vi "Filter Error Codes.vi"   [LabVIEW 2009]
doc: "Filters <b>Error In</b> if matches <b>Error Code to Filter</b>. An <b>Upstream Error</b> can be optionally merged with the resulting filtered error."
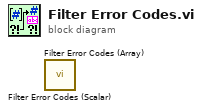
[diagram p0: block diagram]
diagram:
  n1 = call "Filter Error Codes (Scalar).vi"() -> ()  [unwired: 9 in, 3 out]
  n2 = call "Filter Error Codes (Array).vi"() -> ()  [unwired: 9 in, 3 out]
